vi "Simulation.vi"(4 "Modo Simulação":bool, 6 "Tempo de Simulação":dbl, 7 "End":bool, 9 "set_vel":dbl, 10 "Mp":dbl, 11 "read_vel":dbl) -> (0 "erro de estado estacionário":dbl, 1 "Tempo de acomodação":dbl, 2 "Tempo de subida":dbl, 3 "Máximo Overshoot":dbl, 5 "Boolean":bool)   [LabVIEW 2018]
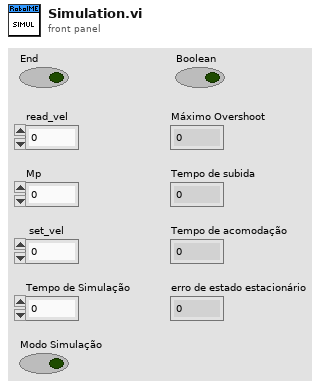
[diagram p1: front panel]
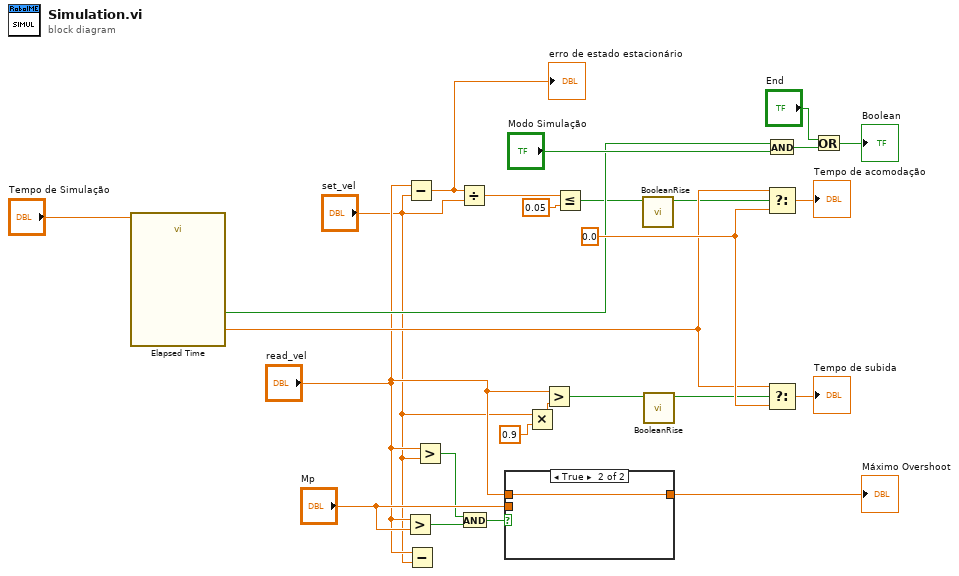
[diagram p0: block diagram]
diagram:
  w24 = 0.0 ("f")
  n1 = call "Elapsed Time"("Time Target (s)"="Tempo de Simulação") -> ("Elapsed Time (s)"=w10:dbl, "Time has Elapsed"=w14:bool)  [unwired: 11 in, 6 out]
  n2 = Greater?(x="read_vel", y="Mp") -> (0:w19:bool)
  n3 = Subtract(x="read_vel", y="set_vel") -> (x-y=w26:dbl)
  "erro de estado estacionário" <- w26
  n4 = Subtract(x="read_vel", y="set_vel") -> ()  [unwired: 1 out]
  n5 = Greater?(x="read_vel", y="set_vel") -> (0:w6:bool)
  n6 = Divide(x=w26, y="set_vel") -> (x/y=w22:dbl)
  n7 = And(x=w6, y=w19) -> (x .and. y?=w18:bool)
  n8 = case shown="True" w18 {
    tunnel: [w27 w28] -> w17
    tunnel: "read_vel" -> [_ w28]
    tunnel: "Mp" -> [w27 _]
    frame False {
    }
    frame True {
    }
  }
  "Máximo Overshoot" <- w17
  n9 = Multiply(x="set_vel", y=0.9) -> (x*y=w3:dbl)
  n10 = Greater?(x="read_vel", y=w3) -> (0:w2:bool)
  n11 = Less Or Equal?(x=w22, y=0.05) -> (x <= y?=w9:bool)
  n12 = call "BooleanRise.vi"("Test Mode On"=w9) -> ("Boolean"=w8:bool)  [unwired: 10 in]
  n13 = call "BooleanRise.vi"("Test Mode On"=w2) -> ("Boolean"=w7:bool)  [unwired: 10 in]
  n14 = And(x=w14, y="Modo Simulação") -> (x .and. y?=w16:bool)
  n15 = Select(t=w10, s=w8, f=w24) -> (s? t:f=→"Tempo de acomodação":dbl)
  n16 = Select(t=w10, s=w7, f=w24) -> (s? t:f=→"Tempo de subida":dbl)
  n17 = Or(x="End", y=w16) -> (x .or. y?=→"Boolean":bool)
